vi "FromXML.vi"(6 "error in":errorcluster, 8 "TestCase element":refnum<k20>) -> (0 "error out":errorcluster, 4 "TestCase out":refnum<class "TestCase.lvclass">)   [LabVIEW 2014, in "TestCase.lvclass"]
uses:
  TestCase.lvclass
  TestCase.lvclass/TestCase.ctl
  <vilib>/xml/NI_XML.lvlib
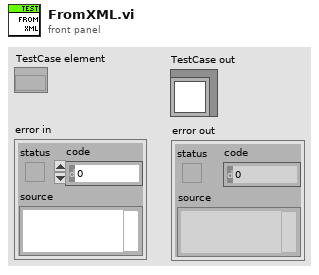
[diagram p1: front panel]
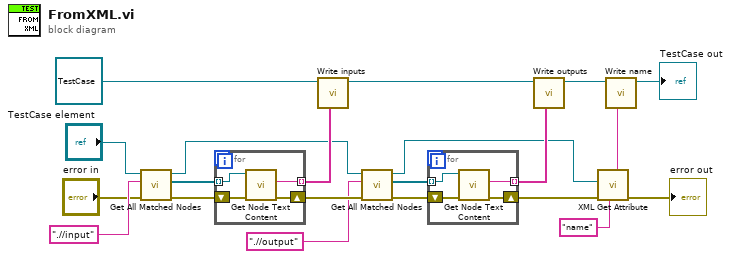
[diagram p0: block diagram]
diagram:
  n1 = call <vilib>:"Get All Matched Nodes.vi"("error in (no error)"="error in", "XPath expression"=".//input", "node in"="TestCase element") -> ("error out"=w18:errorcluster, "node result array"=w19:refnum<k20>[], "node out"=w11:refnum<k20>)  [unwired: 6 in]
  n2 = for {
    tunnel: w19 -> [w24] mode=indexing
    shift-right: [w23] -> w13
    shift-left: w18 -> [w25]
    tunnel: [w22] -> w16 mode=indexing
    n3 = call <vilib>:"Get Node Text Content.vi"("error in (no error)"=w25, "node in"=w24) -> ("error out"=w23:errorcluster, "node text"=w22:string)  [unwired: 7 in, 1 out]
  }
  n4 = call "Write inputs.vi"("inputs"=w16, "TestCase in"=refnum<class "TestCase.lvclass"> refnum) -> ("TestCase out"=w9:refnum<class "TestCase.lvclass">)  [unwired: 7 in]
  n5 = call <vilib>:"Get All Matched Nodes.vi"("error in (no error)"=w13, "XPath expression"=".//output", "node in"=w11) -> ("error out"=w15:errorcluster, "node result array"=w14:refnum<k20>[], "node out"=w6:refnum<k20>)  [unwired: 6 in]
  n6 = for {
    tunnel: w14 -> [w28] mode=indexing
    shift-right: [w27] -> w7
    shift-left: w15 -> [w29]
    tunnel: [w26] -> w8 mode=indexing
    n7 = call <vilib>:"Get Node Text Content.vi"("error in (no error)"=w29, "node in"=w28) -> ("error out"=w27:errorcluster, "node text"=w26:string)  [unwired: 7 in, 1 out]
  }
  n8 = call "Write outputs.vi"("outputs"=w8, "TestCase in"=w9) -> ("TestCase out"=w5:refnum<class "TestCase.lvclass">)  [unwired: 7 in]
  n9 = call "XML Get Attribute.vi"("attribute"="name", "error in"=w7, "node in"=w6) -> ("error out"=→"error out":errorcluster, "value"=w4:string)  [unwired: 4 in, 1 out]
  n10 = call "Write name.vi"("name"=w4, "TestCase in"=w5) -> ("TestCase out"=→"TestCase out":refnum<class "TestCase.lvclass">)  [unwired: 7 in]
